vi "test_IncrementalBuild_SampleProjectSolution.vi"() -> (3 "Pass?":bool)   [LabVIEW 2019, in "Tests.SolutionBuilder.lvlib"]
uses:
  Tests.SolutionBuilder.lvlib
  SolutionBuilder/SolutionBuilder.lvclass
panel:
  out "Second build":cluster{"Build spec name":string, "size":i32}[](array[cluster])
  out "First build":cluster{"Build spec name":string, "size":i32}[](array[cluster])
  out "error out":errorcluster
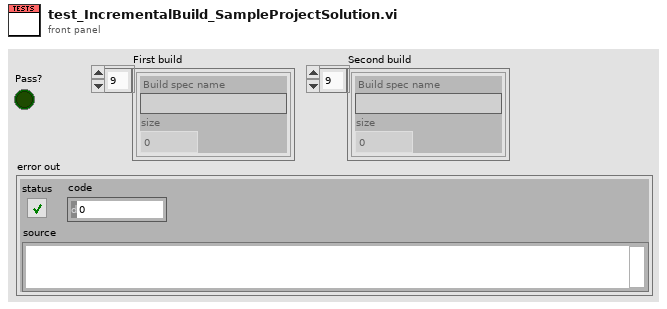
[diagram p1: front panel]
types:
  T1 = typedef "SolutionBuilder.lvlib/BuildManager.lvclass/GeneratedFile.ctl" = map{T2, set{string}}
  T2 = typedef "SolutionBuilder.lvlib/BuildManager.lvclass/BuildProjectInfo.ctl" = cluster{"Project path":string, "Build spec name":string, "Target":string, "Version string":string}
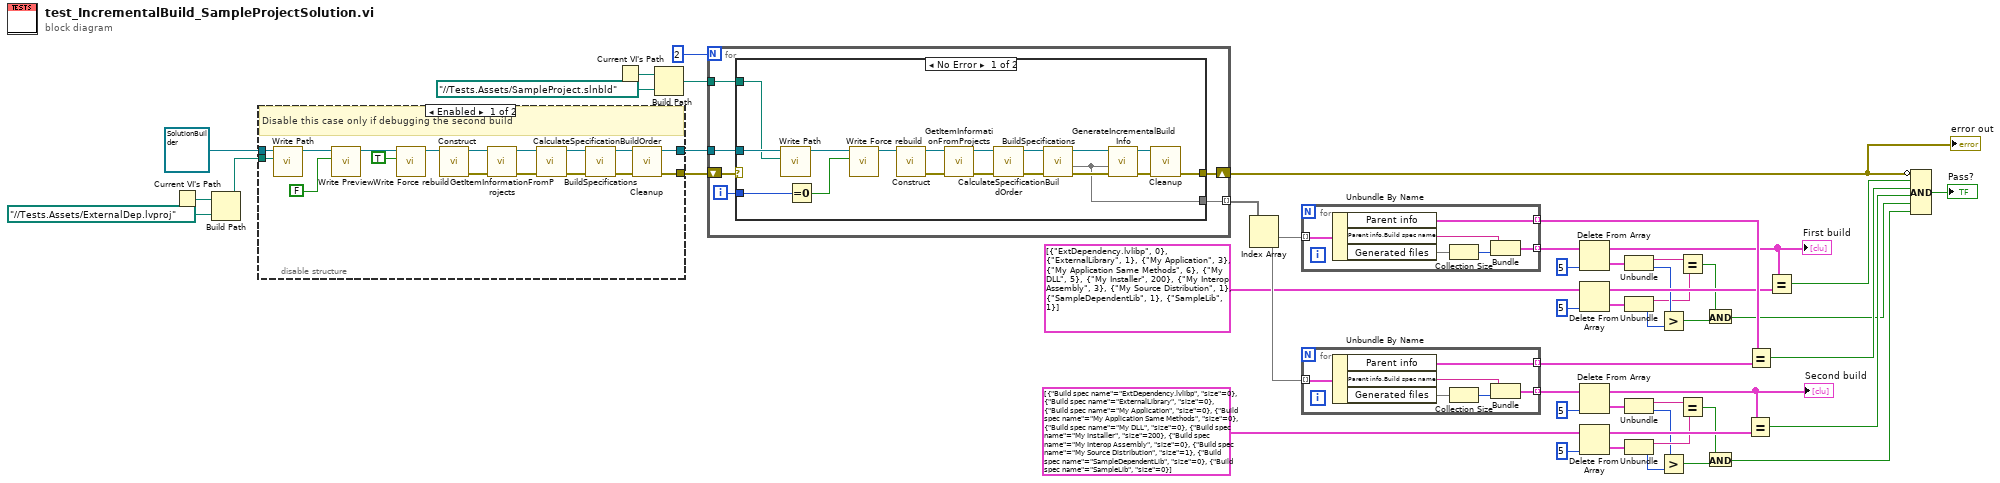
[diagram p0: block diagram]
diagram:
  n1 = Current VI's Path() -> (path=w48:path)
  n2 = Build Path(base path=w48, name or relative path=path "../../Tests.Assets/ExternalDep.lvproj" ("Path")) -> (appended path=w46:path)
  n3 = disable-structure shown="Enabled" {
    disable-tunnel: refnum<class "SolutionBuilder.lvclass"> refnum ("SolutionBuilder in") -> [w67 w68]
    disable-tunnel: w46 -> [w63 _]
    disable-tunnel: [w59 w68] -> w45
    disable-tunnel: [w57 _] -> w44
    frame Enabled {
      # "Disable this case only if debugging the second build"
      n4 = call "Write Path.vi"("Path"=w63, "SolutionBuilder in"=w67) -> ("SolutionBuilder out"=w55:refnum<class "SolutionBuilder.lvclass">)  [unwired: 9 in]
      n5 = call "Write Preview.vi"("Preview?"=FALSE, "SolutionBuilder in"=w55) -> ("SolutionBuilder out"=w53:refnum<class "SolutionBuilder.lvclass">)  [unwired: 9 in]
      n6 = call "Write Force rebuild.vi"("Force rebuild"=TRUE, "SolutionBuilder in"=w53) -> ("SolutionBuilder out"=w52:refnum<class "SolutionBuilder.lvclass">)  [unwired: 9 in]
      n7 = call "Construct.vi"("SolutionBuilder in"=w52) -> ("error out"=w62:errorcluster, "SolutionBuilder out"=w66:refnum<class "SolutionBuilder.lvclass">)  [unwired: 9 in]
      n8 = call "GetItemInformationFromProjects.vi"("error in (no error)"=w62, "SolutionBuilder in"=w66) -> ("error out"=w61:errorcluster, "SolutionBuilder out"=w65:refnum<class "SolutionBuilder.lvclass">)  [unwired: 8 in]
      n9 = call "CalculateSpecificationBuildOrder.vi"("error in (no error)"=w61, "SolutionBuilder in"=w65) -> ("error out"=w60:errorcluster, "SolutionBuilder out"=w64:refnum<class "SolutionBuilder.lvclass">)  [unwired: 8 in]
      n10 = call "BuildSpecifications.vi"("error in (no error)"=w60, "SolutionBuilder in"=w64) -> ("error out"=w58:errorcluster, "SolutionBuilder out"=w56:refnum<class "SolutionBuilder.lvclass">)  [unwired: 7 in, 1 out]
      n11 = call "Cleanup.vi"("error in (no error)"=w58, "SolutionBuilder in"=w56) -> ("error out"=w57:errorcluster, "SolutionBuilder out"=w59:refnum<class "SolutionBuilder.lvclass">)  [unwired: 8 in]
    }
    frame Disabled {
    }
  }
  n12 = Current VI's Path() -> (path=w43:path)
  n13 = Build Path(base path=w43, name or relative path=path "../../Tests.Assets/SampleProject.slnbld" ("Path")) -> (appended path=w41:path)
  n14 = for {
    N: 2 -> [_]
    tunnel: w45 -> [w73]
    tunnel: w41 -> [w71]
    shift-right: [w74] -> w50
    shift-left: w44 -> [w72]
    tunnel: [w70] -> w40 mode=indexing
    i -> [w69]
    n15 = case shown="No Error" w72 {
      selector: w72 -> [_ w93]
      tunnel: w73 -> [w86 _]
      tunnel: [w85 w93] -> w74
      tunnel: w71 -> [w84 _]
      tunnel: [w77 _] -> w70
      tunnel: w69 -> [w81 _]
      frame No Error {
        n16 = call "Write Path.vi"("Path"=w84, "SolutionBuilder in"=w86) -> ("SolutionBuilder out"=w83:refnum<class "SolutionBuilder.lvclass">)  [unwired: 9 in]
        n17 = Equal To 0?(x=w81) -> (x = 0?=w80:bool)
        n18 = call "Write Force rebuild.vi"("Force rebuild"=w80, "SolutionBuilder in"=w83) -> ("SolutionBuilder out"=w82:refnum<class "SolutionBuilder.lvclass">)  [unwired: 9 in]
        n19 = call "Construct.vi"("SolutionBuilder in"=w82) -> ("error out"=w90:errorcluster, "SolutionBuilder out"=w87:refnum<class "SolutionBuilder.lvclass">)  [unwired: 9 in]
        n20 = call "GetItemInformationFromProjects.vi"("error in (no error)"=w90, "SolutionBuilder in"=w87) -> ("error out"=w91:errorcluster, "SolutionBuilder out"=w88:refnum<class "SolutionBuilder.lvclass">)  [unwired: 8 in]
        n21 = call "CalculateSpecificationBuildOrder.vi"("error in (no error)"=w91, "SolutionBuilder in"=w88) -> ("error out"=w92:errorcluster, "SolutionBuilder out"=w89:refnum<class "SolutionBuilder.lvclass">)  [unwired: 8 in]
        n22 = call "BuildSpecifications.vi"("error in (no error)"=w92, "SolutionBuilder in"=w89) -> ("error out"=w78:errorcluster, "Generated file"=w77:T1, "SolutionBuilder out"=w79:refnum<class "SolutionBuilder.lvclass">)  [unwired: 7 in]
        n23 = call "GenerateIncrementalBuildInfo.vi"("error in (no error)"=w78, "Generated file"=w77, "SolutionBuilder in"=w79) -> ("error out"=w75:errorcluster, "SolutionBuilder out"=w76:refnum<class "SolutionBuilder.lvclass">)  [unwired: 7 in]
        n24 = call "Cleanup.vi"("error in (no error)"=w75, "SolutionBuilder in"=w76) -> ("error out"=w85:errorcluster)  [unwired: 8 in, 1 out]
      }
      frame Error {
      }
    }
  }
  "error out" <- w50
  n25 = Index Array(array=w40) -> (element #1=w39:T1, element #2=w35:T1)  [unwired: 2 in]
  n26 = for {
    tunnel: w39 -> [w99] mode=indexing
    tunnel: [w98] -> w38 mode=indexing
    tunnel: [w94] -> w21 mode=indexing
    n27 = Unbundle By Name(w99) -> ("Parent info"=w98:T2, "Parent info.Build spec name"=w96:string, "Generated files"=w97:set{string})
    n28 = Collection Size(1:w97) -> (0:w95:i32)
    n29 = Bundle("Build spec name"=w96, "size"=w95) -> (w94:cluster{"Build spec name":string, "size":i32})  [unwired: 1 in]
  }
  n30 = for {
    tunnel: w35 -> [w105] mode=indexing
    tunnel: [w104] -> w34 mode=indexing
    tunnel: [w100] -> w31 mode=indexing
    n31 = Unbundle By Name(w105) -> ("Parent info"=w104:T2, "Parent info.Build spec name"=w102:string, "Generated files"=w103:set{string})
    n32 = Collection Size(1:w103) -> (0:w101:i32)
    n33 = Bundle("Build spec name"=w102, "size"=w101) -> (w100:cluster{"Build spec name":string, "size":i32})  [unwired: 1 in]
  }
  n34 = Delete From Array(array=w21, index=5) -> (deleted portion=w3:cluster{"Build spec name":string, "size":i32}, array with subset deleted=w20:cluster{"Build spec name":string, "size":i32}[])  [unwired: 1 in]
  "First build" <- w20
  n35 = Delete From Array(array=cluster{"Build spec name":string, "size":i32}[] [{"Build spec name"="ExtDependency.lvlibp", "size"=0}, {"Build spec name"="ExternalLibrary", "size"=1}, {"Build spec name"="My Application", "size"=3}, {"Build spec name"="My Application Same Methods", "size"=6}, {"Build spec name"="My DLL", "size"=5}, {"Build spec name"="My Installer", "size"=200}, {"Build spec name"="My Interop Assembly", "size"=3}, {"Build spec name"="My Source Distribution", "size"=1}, {"Build spec name"="SampleDependentLib", "size"=1}, {"Build spec name"="SampleLib", "size"=1}] ("Array"), index=5) -> (deleted portion=w2:cluster{"Build spec name":string, "size":i32}, array with subset deleted=w23:cluster{"Build spec name":string, "size":i32}[])  [unwired: 1 in]
  n36 = Delete From Array(array=w31, index=5) -> (deleted portion=w18:cluster{"Build spec name":string, "size":i32}, array with subset deleted=w19:cluster{"Build spec name":string, "size":i32}[])  [unwired: 1 in]
  "Second build" <- w19
  n37 = Delete From Array(array=cluster{"Build spec name":string, "size":i32}[] [{"Build spec name"="ExtDependency.lvlibp", "size"=0}, {"Build spec name"="ExternalLibrary", "size"=0}, {"Build spec name"="My Application", "size"=0}, {"Build spec name"="My Application Same Methods", "size"=0}, {"Build spec name"="My DLL", "size"=0}, {"Build spec name"="My Installer", "size"=200}, {"Build spec name"="My Interop Assembly", "size"=0}, {"Build spec name"="My Source Distribution", "size"=1}, {"Build spec name"="SampleDependentLib", "size"=0}, {"Build spec name"="SampleLib", "size"=0}] ("Array 2"), index=5) -> (deleted portion=w17:cluster{"Build spec name":string, "size":i32}, array with subset deleted=w26:cluster{"Build spec name":string, "size":i32}[])  [unwired: 1 in]
  n38 = Unbundle(w3) -> ("Build spec name"=w4:string, "size"=w6:i32)
  n39 = Unbundle(w2) -> ("Build spec name"=w5:string, "size"=w7:i32)
  n40 = Unbundle(w18) -> ("Build spec name"=w16:string, "size"=w14:i32)
  n41 = Unbundle(w17) -> ("Build spec name"=w15:string, "size"=w13:i32)
  n42 = Greater?(x=w6, y=w7) -> (0:w9:bool)
  n43 = Greater?(x=w14, y=w13) -> (0:w11:bool)
  n44 = Equal?(x=w4, y=w5) -> (x = y?=w8:bool)
  n45 = Equal?(x=w16, y=w15) -> (x = y?=w12:bool)
  n46 = And(x=w8, y=w9) -> (x .and. y?=w1:bool)
  n47 = And(x=w12, y=w11) -> (x .and. y?=w10:bool)
  n48 = Equal?(x=w19, y=w26) -> (x = y?=w30:bool)
  n49 = Equal?(x=w38, y=w34) -> (x = y?=w33:bool)
  n50 = Equal?(x=w20, y=w23) -> (x = y?=w32:bool)
  n51 = Compound Arithmetic op=AND(invert w50, w32, w33, w30, w1, w10) -> (→"Pass?":bool)
